vi "Main_dequeue.vi"(8 "error in (no error)":errorcluster, 11 "Queue in":refnum<queue>) -> (0 "error out":errorcluster, 2 "Cmd":string, 3 "Queue out":refnum<queue>)   [LabVIEW 2016]
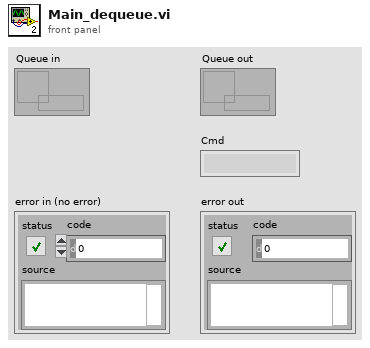
[diagram p1: front panel]
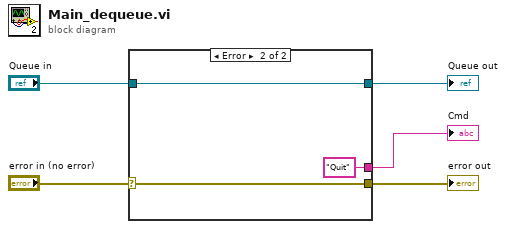
[diagram p0: block diagram]
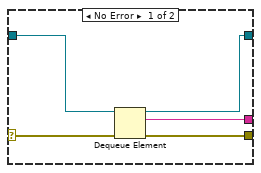
[diagram p2: hidden frame]
diagram:
  n1 = case shown="Error" "error in (no error)" {
    selector: "error in (no error)" -> [w6 w12]
    tunnel: [w10 "Quit" ("Cmd")] -> w5
    tunnel: [w9 w11] -> w4
    tunnel: [w8 w12] -> w3
    tunnel: "Queue in" -> [w7 w11]
    frame No Error {
      n2 = Dequeue Element(queue=w7, error in (no error)=w6) -> (queue out=w9:refnum<queue>, element=w10:string, error out=w8:errorcluster)  [unwired: 1 in, 1 out]
    }
    frame Error {
    }
  }
  "Cmd" <- w5
  "Queue out" <- w4
  "error out" <- w3
